vi "INTERCAMBIADOR DE CALOR_original.vi"() -> ()   [LabVIEW 2017]
uses:
  <vilib>/Platform/TimedLoop/XDataNode/timing_clust.ctl
  <vilib>/Platform/TimedLoop/XDataNode/nitl_modes.ctl
  <vilib>/Platform/TimedLoop/XDataNode/wakeup.ctl
  <vilib>/platform/TimedLoop/XDataNode/XDataNode.xnode
  <vilib>/Platform/TimedLoop/XDataNode/XDNodeRunTimeDep.lvlib
panel:
  out "XY Graph 4":cluster{dbl[], sgl[]}[](graph)
  out "XY Graph 3":cluster{dbl[], sgl[]}(graph)
  out "XY Graph 2":cluster{dbl[], sgl[]}(graph)
  out "Period":i64
  in  "% Apertura de válvula 2":dbl(slide) scale=0.0..6.7e-06
  out "time":dbl
  out "FC":dbl
  in  "% Apertura de válvula":dbl(slide) scale=0.0..2e-05
  in  "Tci":dbl
  in  "Thi":dbl
  out "FH":dbl
  out "tco":sgl
  out "tho":sgl
  out "Delta":sgl
  in  "Stop Button":bool
  # "INTERCAMBIADOR DE CALOR"
  # "TCO"
  # "THO"
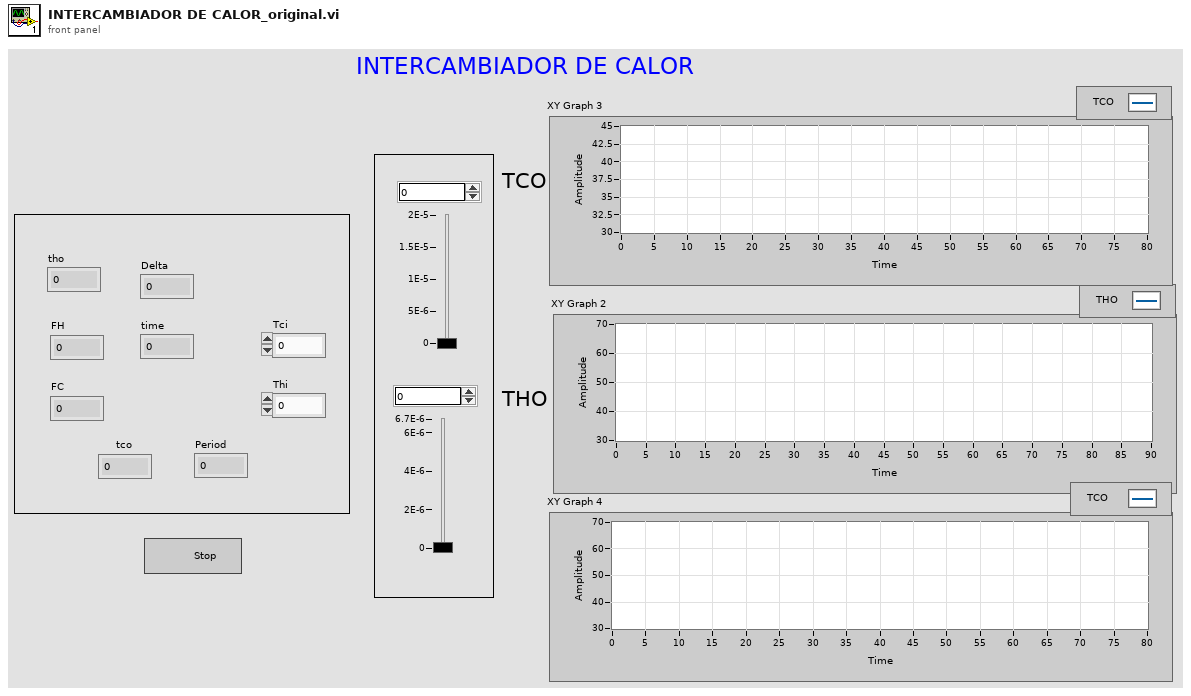
[diagram p1: front panel]
types:
  T1 = typedef "XDNodeRunTimeDep.lvlib/timing_clust.ctl" = cluster{"Expected End [f-1]":u64, "Actual End [f-1]":u64, "Finished Late? [f-1]":bool, "Expected End [i-1]":u64, "Actual End [i-1]":u64, "Finished Late? [i-1]":bool, "Expected Start [i]":u64, "Actual Start [i]":u64, "Expected Start [f]":u64, "Actual Start [f]":u64, "Source Name":string, "Structure Name":string, "Period":i64, "Deadline":i64, "Offset":i64, "Start":i64, "Priority":i32, "Timeout":i32, "Mode":T2, "Wakeup Reason":T3, "Error":errorcluster, "Source Type":string, "Secondary Source Type":string, "Global End Time":u64, "Global Start Time":u64, "Frame Duration":u64, "Iteration Duration":u64, "Assigned CPU":i32, "I/O Scan Engine Mode":u32}
  T2 = typedef "XDNodeRunTimeDep.lvlib/nitl_modes.ctl" = enum32{"No Change", "Process missed periods, maintain original phase", "Discard missed periods, maintain original phase", "Process missed periods, ignore original phase", "Discard missed periods, ignore original phase"}
  T3 = typedef "XDNodeRunTimeDep.lvlib/wakeup.ctl" = enum32{"Normal", "Aborted", "Asynchronous wakeup", "Timing source error", "Timed loop error", "Timeout"}
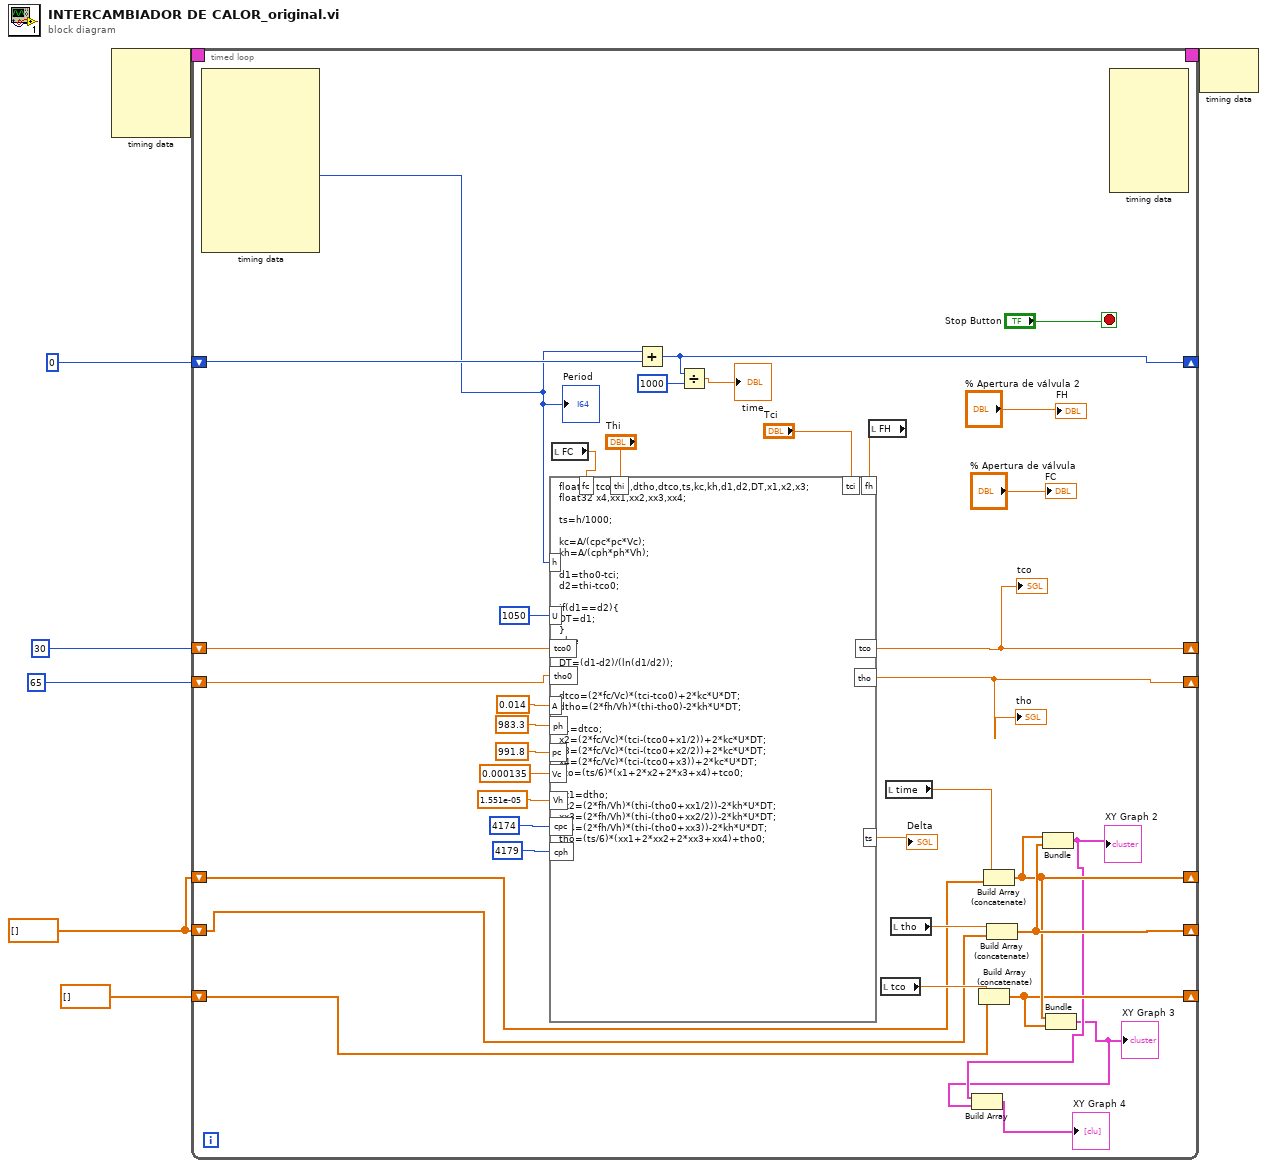
[diagram p0: block diagram]
diagram:
  w1 = sgl[] []
  n1 = node-c288() -> (w5:T1)  [unwired: 4 in]
  n2 = timed-loop {
    shift-right: [w35] -> _
    shift-left: 30 -> [w34]
    shift-right: [w21] -> _
    shift-left: 65 -> [w33]
    timing: w5 -> [_]
    timing-out: [_] -> w4
    shift-right: [w26] -> _
    shift-left: i64 0 -> [w25]
    shift-right: [w12] -> _
    shift-left: w1 -> [w16]
    shift-right: [w13] -> _
    shift-left: w1 -> [w15]
    shift-right: [w11] -> _
    shift-left: sgl[] [] -> [w14]
    stop <- "Stop Button" stop-if-true
    n3 = node-c288() -> (w24:i64)  [unwired: 1 in, 10 out]
    "Period" <- w24
    n4 = local read "FC"() -> (w22:dbl)
    n5 = Add(x=w24, y=w25) -> (x+y=w26:i64)
    n6 = Divide(x=w26, y=i64 1000) -> (x/y=→"time":dbl)
    n7 = local read "FH"() -> (w32:dbl)
    n8 = formula code="float32 tco,tho,dtho,dtco,ts,kc,kh,d1,d2,DT,x1,x2,x3;\nfloat32 x4,xx1,xx2,xx3,xx4;\n\nts=h/1000;\n\nkc=A/(cpc*pc*Vc);\nkh=A/(cph*ph*Vh);\n\nd1=tho0-tci;\nd2=thi-tco0;\n\nif(d1==d2){\nDT=d1;\n}\nelse\n{\nDT=(d1-d2)/(ln(d1/d2));\n}\n\ndtco=(2*fc/Vc)*(tci-tco0)+2*kc*U*DT;\ndtho=(2*fh/Vh)*(thi-tho0)-2*kh*U*DT;\n\nx1=dtco;\nx2=(2*fc/Vc)*(tci-(tco0+x1/2))+2*kc*U*DT;\nx3=(2*fc/Vc)*(tci-(tco0+x2/2))+2*kc*U*DT;\nx4=(2*fc/Vc)*(tci-(tco0+x3))+2*kc*U*DT;\ntco=(ts/6)*(x1+2*x2+2*x3+x4)+tco0;\n\nxx1=dtho;\nxx2=(2*fh/Vh)*(thi-(tho0+xx1/2))-2*kh*U*DT;\nxx3=(2*fh/Vh)*(thi-(tho0+xx2/2))-2*kh*U*DT;\nxx4=(2*fh/Vh)*(thi-(tho0+xx3))-2*kh*U*DT;\ntho=(ts/6)*(xx1+2*xx2+2*xx3+xx4)+tho0;"("tco0"=w34, "tho0"=w33, "h"=w24, "fc"=w22, "thi"="Thi", "tci"="Tci", "A"=0.014, "ph"=983.3, "pc"=991.8, "Vc"=0.000135, "Vh"=1.551e-05, "cpc"=4174, "cph"=4179, "U"=1050, "fh"=w32) -> ("tco"=w35:sgl, "tho"=w21:sgl, "ts"=→"Delta":sgl)
    "tho" <- w21
    "tco" <- w35
    n9 = local read "tco"() -> (w17:sgl)
    n10 = local read "time"() -> (w19:dbl)
    n11 = local read "tho"() -> (w18:sgl)
    n12 = Build Array (concatenate)(w17, w14) -> (w11:sgl[])
    n13 = Build Array (concatenate)(w19, w16) -> (w12:dbl[])
    n14 = Build Array (concatenate)(w18, w15) -> (w13:sgl[])
    n15 = Bundle(w12, w13) -> (w10:cluster{dbl[], sgl[]})  [unwired: 1 in]
    "XY Graph 2" <- w10
    n16 = Bundle(w12, w11) -> (w9:cluster{dbl[], sgl[]})  [unwired: 1 in]
    "XY Graph 3" <- w9
    n17 = Build Array(w10, w9) -> (→"XY Graph 4":cluster{dbl[], sgl[]}[])
    n18 = node-c288() -> ()  [unwired: 7 in, 1 out]
    "FH" <- "% Apertura de válvula 2"
    "FC" <- "% Apertura de válvula"
  }
  n19 = node-c288(w4) -> ()  [unwired: 1 out]
